vi "FUG-HCN.setprecision 1.vi"(0 "i ref in":refnum<vi>, 3 "ms timeout (100)":i32=100, 5 "error in (no error)":errorcluster) -> (14 "i ref out":refnum<vi>, 16 "Precision":dbl format="%.2f", 17 "timed out":bool, 19 "error out":errorcluster)   [LabVIEW 2014, in "FUG-HCN.lvlib"]
uses:
  FUG-HCN.lvlib
  CSCore/BaseProcess/BaseProcess.lvlib
  CSCore/CSObj/CSObj.lvlib
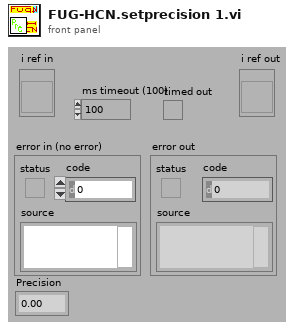
[diagram p1: front panel]
types:
  T1 = typedef "BaseProcess.lvlib/BaseProcess.i attribute.ctl" = cluster{"EventStatus":string, "EventError":i32, "PresetEvtWatchD":i32, "PresetPdcWatchD":i32, "EventTimeout":i32, "PeriodicInterval":i32, "Interface":string[], "Address":string[], "Special":string[], "PeriodicError":i32, "PeriodicStatus":string, "SuperProc":string, "Descriptors":T2[], "CaseRef":refnum<vi>, "PdcRef":refnum<vi>, "Thread Ref":refnum<vi>, "eventErrorID":i32, "eventStatusID":i32, "periodicErrorID":i32, "periodicStatusID":i32, "pdcCtrID":i32}
  T2 = typedef "BaseProcess.lvlib/BaseProcess.descriptor definition.ctl" = cluster{"selector":string, "descriptor":T3}
  T3 = typedef "BaseProcess.lvlib/BaseProcess.descriptor string definition.ctl" = string
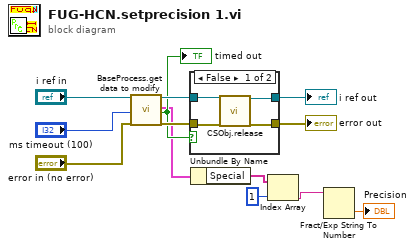
[diagram p0: block diagram]
diagram:
  n1 = call "BaseProcess.get data to modify.vi"("i ref in"="i ref in", "ms timeout (10000)"="ms timeout (100)", "error in (no error)"="error in (no error)") -> ("i ref out"=w9:refnum<vi>, "i attribute"=w5:T1, "timed out"=w6:bool, "error out"=w8:errorcluster)  [unwired: 13 in]
  "timed out" <- w6
  n2 = case shown="False" w6 {
    tunnel: [w15 w18] -> w11
    tunnel: [w16 w19] -> w10
    tunnel: w9 -> [w17 w19]
    tunnel: w8 -> [w14 w18]
    frame False {
      n3 = call "CSObj.release.vi"("i ref in"=w17, "error in (no error)"=w14) -> ("i ref out"=w16:refnum<vi>, "error out"=w15:errorcluster)  [unwired: 16 in]
    }
    frame True {
    }
  }
  "error out" <- w11
  "i ref out" <- w10
  n4 = Unbundle By Name(w5) -> ("Special"=w3:string[])
  n5 = Index Array(array=w3, index=1) -> (element=w4:string)
  n6 = Fract/Exp String To Number(string=w4) -> (number=→"Precision":dbl)  [unwired: 3 in, 1 out]
